vi "CSDB_Config.set string values.vi"(3 "Type":string, 4 "AttributeName":string, 8 "Values in":string[](array[string]), 10 "InstanceNames in":string[](array[string])) -> (16 "Values out":string[](array[string]))   [LabVIEW 2014, in "CSDB_Config.lvlib"]
doc: "sets string values of attribute data"
uses:
  CSDB_Config.lvlib
panel:
  in  "cancel":bool
  in  "apply":bool
  in  "Table":i32[](listbox)
  in  "ADD an INDEX":enum32{"numerical", "alphabet"}(tab)
  in  "starting number":dbl
  in  "starting letter":string
  in  "suf":bool
  in  "pref":bool
  in  "Set Values":string
  in  "done":bool
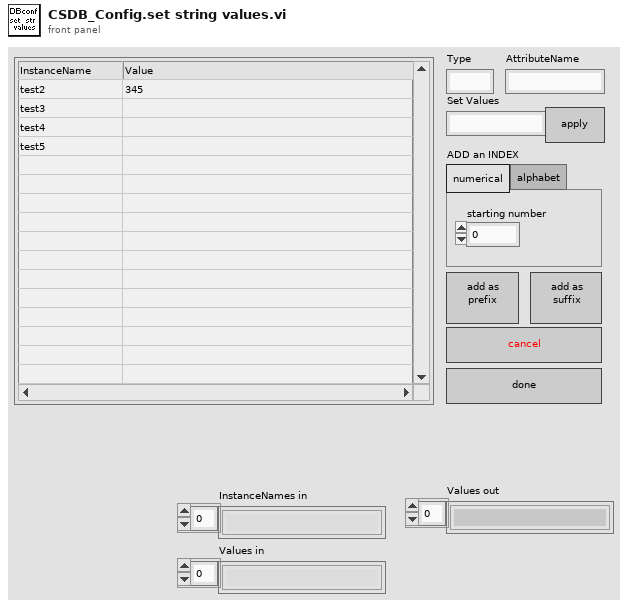
[diagram p1: front panel]
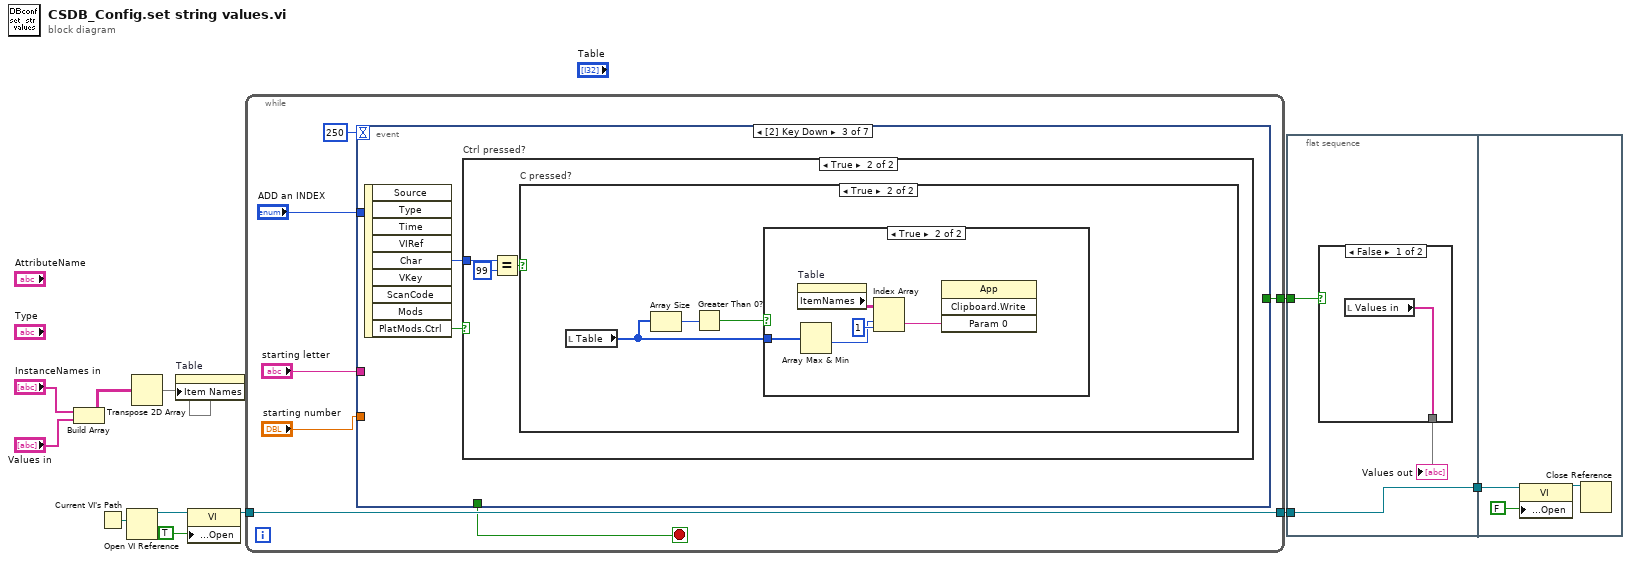
[diagram p0: block diagram]
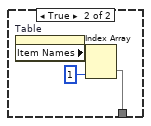
[diagram p2: hidden frame]
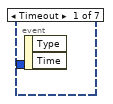
[diagram p3: hidden frame]
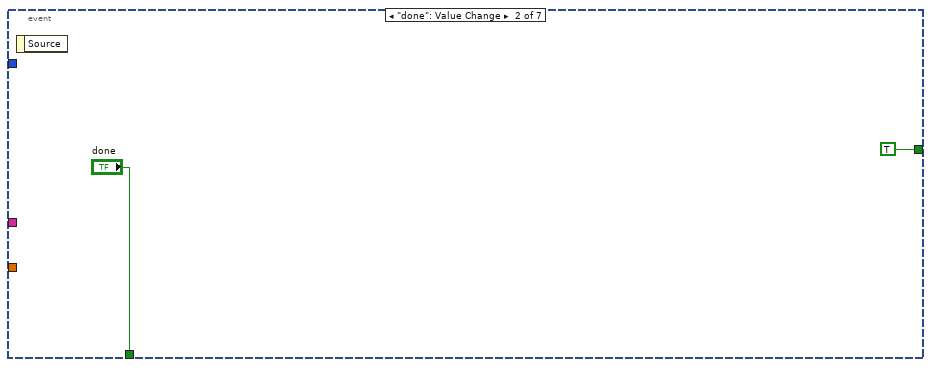
[diagram p4: hidden frame]
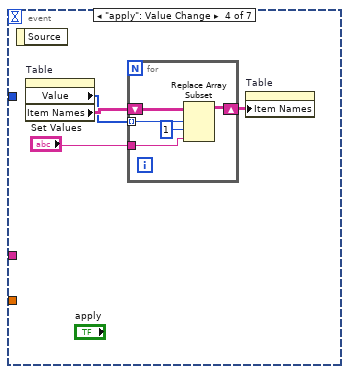
[diagram p8: hidden frame]
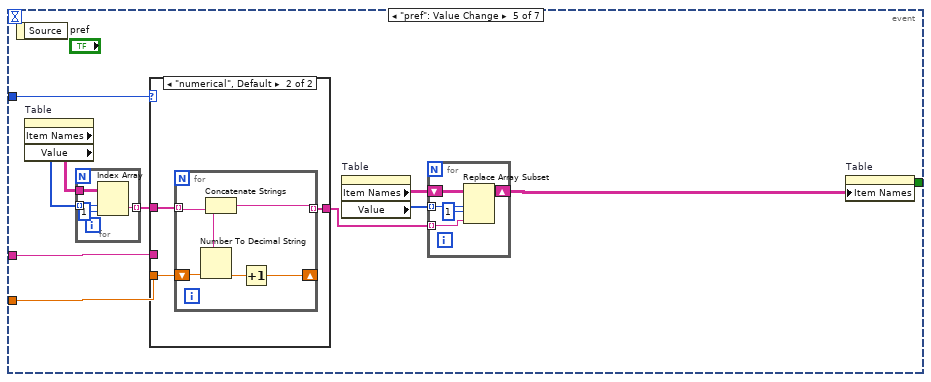
[diagram p9: hidden frame]
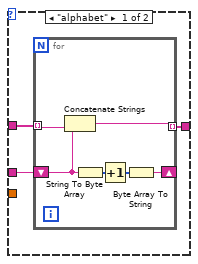
[diagram p10: hidden frame]
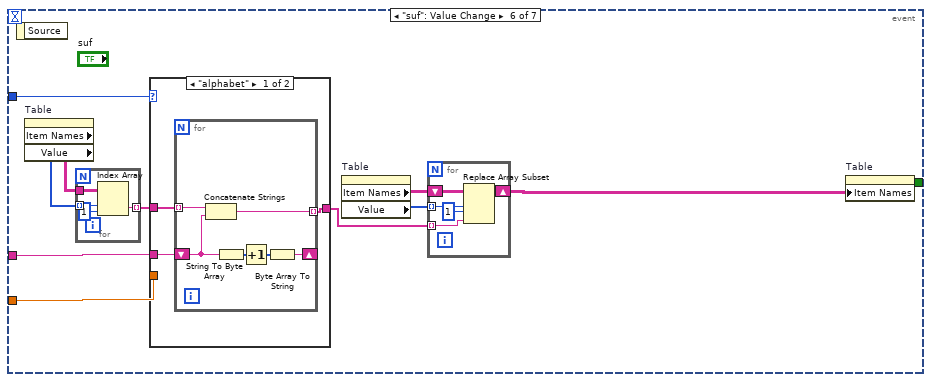
[diagram p11: hidden frame]
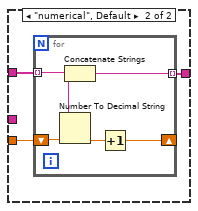
[diagram p12: hidden frame]
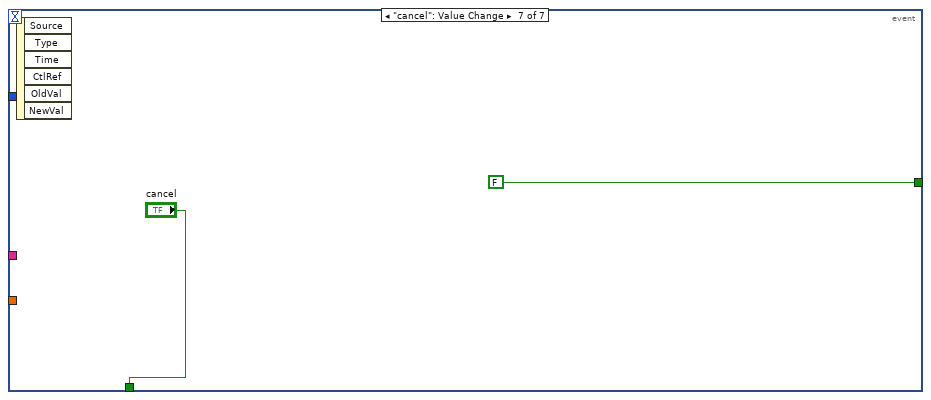
[diagram p13: hidden frame]
diagram:
  n1 = Build Array("InstanceNames in", "Values in") -> (w5:string[][])
  n2 = Current VI's Path() -> (path=w11:path)
  n3 = Open VI Reference(vi path=w11) -> (vi reference=w10:refnum<vi>)  [unwired: 5 in, 1 out]
  n4 = Transpose 2D Array(2D array=w5) -> (transposed array=w4:string[][])
  n5 = property on="Table" class="MCListbox (strict)"("Item Names"=w4) -> ()  [unwired: 2 in, 2 out]
  n6 = property class="VI"(reference=w10, "Front Panel Window:Open"=TRUE) -> (reference out=w8:refnum<vi>)  [unwired: 1 in, 1 out]
  n7 = while {
    tunnel: [w18] -> w3
    tunnel: w8 -> [w18]
    tunnel: [w13] -> w1
    stop <- w17 stop-if-true
    n8 = event shown="[2] Key Down" {
      selector: _ -> [_ _ _ _ _ _ _]
      dyn-events: _ -> [_ _ _ _ _ _ _]
      timeout: 250 -> [_ _ _ _ _ _ _]
      tunnel: [_ "done" _ _ _ _ "cancel"] -> w17
      tunnel: "ADD an INDEX" -> [_ _ _ _ w52 w88 _]
      tunnel: "starting letter" -> [_ _ _ _ w49 w85 _]
      tunnel: "starting number" -> [_ _ _ _ w48 w84 _]
      tunnel: [_ TRUE _ _ _ _ FALSE] -> w13
      event Timeout {
        n9 = event-data() -> ()  [unwired: 1 in, 2 out]
      }
      event "done": Value Change {
        n10 = event-data() -> ()  [unwired: 1 in, 1 out]
      }
      event Key Down {
        n11 = event-data() -> ("Char"=w21:i16, "PlatMods.Ctrl"=w22:bool)  [unwired: 1 in, 7 out]
        n12 = case "Ctrl pressed?" shown="True" w22 {
          tunnel: w21 -> [_ w23]
          frame False {
          }
          frame True {
            n13 = Equal?(x=w23, y=i16 99) -> (x = y?=w24:bool)
            n14 = case "C pressed?" shown="True" w24 {
              frame False {
              }
              frame True {
                n15 = local read "Table"() -> (w28:i32[])
                n16 = Array Size(array=w28) -> (size(s)=w27:i32)
                n17 = Greater Than 0?(x=w27) -> (x > 0?=w26:bool)
                n18 = case shown="True" w26 {
                  tunnel: w28 -> [_ w30]
                  frame False {
                  }
                  frame True {
                    n19 = property on="Table" class="MCListbox (strict)"() -> ("ItemNames"=w33:string[][])  [unwired: 2 in, 2 out]
                    n20 = Array Max & Min(array=w30) -> (min value=w29:i32)  [unwired: 3 out]
                    n21 = Index Array(array=w33, index (row)=w29, index (col)=1 ("disabled index (col)")) -> (element=w32:string)
                    n22 = invoke class="App" method="Clipboard.Write"("Param 0"=w32) -> ()  [unwired: 3 in, 4 out]
                  }
                }
              }
            }
          }
        }
      }
      event "apply": Value Change {
        n23 = event-data() -> ()  [unwired: 1 in, 1 out]
        n24 = property on="Table" class="MCListbox (strict)"() -> ("Value"=w36:i32[], "Item Names"=w37:string[][])  [unwired: 2 in, 2 out]
        n25 = for {
          tunnel: "Set Values" -> [w39]
          tunnel: w36 -> [w41] mode=indexing
          shift-right: [w38] -> w35
          shift-left: w37 -> [w42]
          n26 = Replace Array Subset(array=w42, new element=w39, index (row)=w41, index (col)=1 ("disabled index (col)")) -> (w38:string[][])
        }
        n27 = property on="Table" class="MCListbox (strict)"("Item Names"=w35) -> ()  [unwired: 2 in, 2 out]
      }
      event "pref": Value Change {
        n28 = event-data() -> ()  [unwired: 1 in, 1 out]
        n29 = property on="Table" class="MCListbox (strict)"() -> ("Item Names"=w51:string[][], "Value"=w47:i32[])  [unwired: 2 in, 2 out]
        n30 = for {
          tunnel: w51 -> [w61]
          tunnel: w47 -> [w60] mode=indexing
          tunnel: [w58] -> w50 mode=indexing
          n31 = Index Array(array=w61, index (row)=w60, index (col)=1 ("disabled index (col)")) -> (element=w58:string)
        }
        n32 = case shown="\"numerical\", Default" w52 {
          tunnel: w50 -> [w64 w73]
          tunnel: w49 -> [w63 _]
          tunnel: w48 -> [_ w72]
          tunnel: [w62 w71] -> w44
          frame "alphabet" {
            n33 = for {
              tunnel: [w70] -> w62 mode=indexing
              shift-right: [w66] -> _
              shift-left: w63 -> [w67]
              tunnel: w64 -> [w65] mode=indexing
              n34 = Concatenate Strings(w67, w65) -> (w70:string)
              n35 = String To Byte Array(string=w67) -> (unsigned byte array=w68:u8[])
              n36 = Increment(x=w68) -> (x+1=w69:u8[])
              n37 = Byte Array To String(unsigned byte array=w69) -> (string=w66:string)
            }
          }
          frame "numerical", Default {
            n38 = for {
              tunnel: [w78] -> w71 mode=indexing
              shift-right: [w74] -> _
              shift-left: w72 -> [w75]
              tunnel: w73 -> [w77] mode=indexing
              n39 = Number To Decimal String(number=w75) -> (decimal integer string=w76:string)  [unwired: 1 in]
              n40 = Concatenate Strings(w76, w77) -> (w78:string)
              n41 = Increment(x=w75) -> (x+1=w74:dbl)
            }
          }
        }
        n42 = property on="Table" class="MCListbox (strict)"() -> ("Item Names"=w46:string[][], "Value"=w45:i32[])  [unwired: 2 in, 2 out]
        n43 = for {
          tunnel: w45 -> [w56] mode=indexing
          tunnel: w44 -> [w54] mode=indexing
          shift-right: [w53] -> w43
          shift-left: w46 -> [w57]
          n44 = Replace Array Subset(array=w57, new element=w54, index (row)=w56, index (col)=1 ("disabled index (col)")) -> (w53:string[][])
        }
        n45 = property on="Table" class="MCListbox (strict)"("Item Names"=w43) -> ()  [unwired: 2 in, 2 out]
      }
      event "suf": Value Change {
        n46 = event-data() -> ()  [unwired: 1 in, 1 out]
        n47 = property on="Table" class="MCListbox (strict)"() -> ("Item Names"=w87:string[][], "Value"=w83:i32[])  [unwired: 2 in, 2 out]
        n48 = for {
          tunnel: w87 -> [w97]
          tunnel: w83 -> [w96] mode=indexing
          tunnel: [w94] -> w86 mode=indexing
          n49 = Index Array(array=w97, index (row)=w96, index (col)=1 ("disabled index (col)")) -> (element=w94:string)
        }
        n50 = case shown="\"alphabet\"" w88 {
          tunnel: w86 -> [w100 w109]
          tunnel: w85 -> [w99 _]
          tunnel: w84 -> [_ w108]
          tunnel: [w98 w107] -> w80
          frame "alphabet" {
            n51 = for {
              tunnel: [w106] -> w98 mode=indexing
              shift-right: [w103] -> _
              shift-left: w99 -> [w101]
              tunnel: w100 -> [w102] mode=indexing
              n52 = Concatenate Strings(w102, w101) -> (w106:string)
              n53 = String To Byte Array(string=w101) -> (unsigned byte array=w104:u8[])
              n54 = Increment(x=w104) -> (x+1=w105:u8[])
              n55 = Byte Array To String(unsigned byte array=w105) -> (string=w103:string)
            }
          }
          frame "numerical", Default {
            n56 = for {
              tunnel: [w114] -> w107 mode=indexing
              shift-right: [w112] -> _
              shift-left: w108 -> [w113]
              tunnel: w109 -> [w111] mode=indexing
              n57 = Number To Decimal String(number=w113) -> (decimal integer string=w110:string)  [unwired: 1 in]
              n58 = Concatenate Strings(w111, w110) -> (w114:string)
              n59 = Increment(x=w113) -> (x+1=w112:dbl)
            }
          }
        }
        n60 = property on="Table" class="MCListbox (strict)"() -> ("Item Names"=w82:string[][], "Value"=w81:i32[])  [unwired: 2 in, 2 out]
        n61 = for {
          tunnel: w81 -> [w92] mode=indexing
          tunnel: w80 -> [w90] mode=indexing
          shift-right: [w89] -> w79
          shift-left: w82 -> [w93]
          n62 = Replace Array Subset(array=w93, new element=w90, index (row)=w92, index (col)=1 ("disabled index (col)")) -> (w89:string[][])
        }
        n63 = property on="Table" class="MCListbox (strict)"("Item Names"=w79) -> ()  [unwired: 2 in, 2 out]
      }
      event "cancel": Value Change {
        n64 = event-data() -> ()  [unwired: 1 in, 6 out]
      }
    }
  }
  n65 = flat-sequence {
    tunnel: w3 -> [w118]
    tunnel: [w118] -> w2
    tunnel: w1 -> [w117]
    tunnel: w2 -> [w124]
    frame #0 {
      n66 = case shown="False" w117 {
        tunnel: [w120 w121] -> w119
        frame False {
          n67 = local read "Values in"() -> (w120:string[])
        }
        frame True {
          n68 = property on="Table" class="MCListbox (strict)"() -> ("Item Names"=w123:string[][])  [unwired: 2 in, 2 out]
          n69 = Index Array(array=w123, index (col)=1 ("disabled index (col)")) -> (element=w121:string[])  [unwired: 1 in]
        }
      }
      "Values out" <- w119
    }
    frame #1 {
      n70 = property class="VI"(reference=w124, "Front Panel Window:Open"=FALSE) -> (reference out=w126:refnum<vi>)  [unwired: 1 in, 1 out]
      n71 = Close Reference(reference=w126) -> ()  [unwired: 1 in, 1 out]
    }
  }
